vi "uSubscription IsAlive.vi"(8 "error in (no error)":errorcluster, 11 "uSubscription in":refnum<class "uSubscription.lvclass">) -> (0 "error out":errorcluster, 2 "Is Alive?":bool)   [LabVIEW 2023, in "uLib.lvlib" / "uSubscription.lvclass"]
uses:
  uSubscription.lvclass
  uSubscription.lvclass/uSubscription.ctl
  uTransport/uTransport/uTransport.lvclass
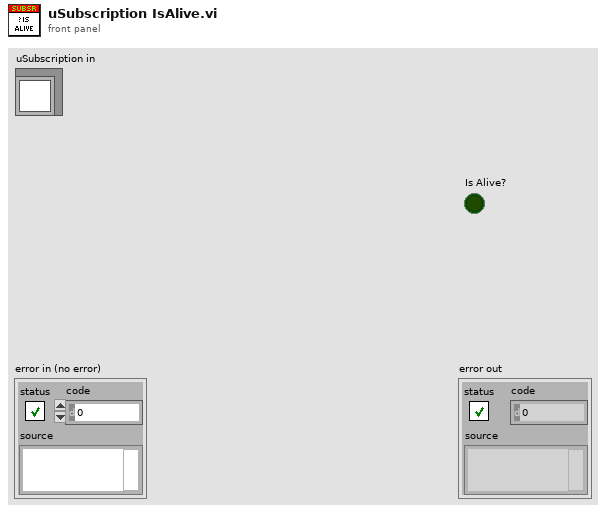
[diagram p1: front panel]
types:
  T1 = typedef "uLib.lvlib/uSubscription.lvclass/TypeDef_uSubscriptionPrivateData.ctl" = cluster{"Destination CMD":string, "uNotifyMode":refnum<class "uNotifyMode.lvclass">, "Destination uTransport":refnum<class "uTransport.lvclass">}
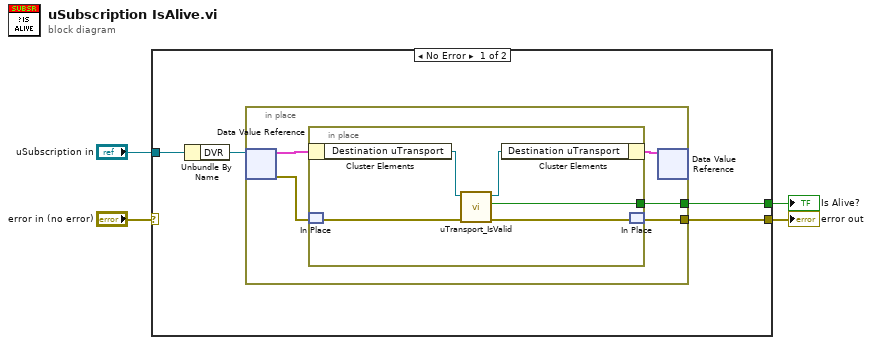
[diagram p0: block diagram]
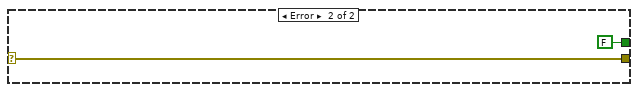
[diagram p2: hidden frame]
diagram:
  n1 = case shown="No Error" "error in (no error)" {
    selector: "error in (no error)" -> [_ w20]
    tunnel: [w8 w20] -> w4
    tunnel: [w7 FALSE ("IsValid?")] -> w3
    tunnel: "uSubscription in" -> [w6 _]
    frame No Error {
      n2 = Unbundle By Name(w6) -> ("DVR"=w5:refnum<data-value>)
      n3 = in-place {
        in-place-border: [w10] -> w8
        in-place-border: [w13] -> w7
        n4 = in-place-dvr #1(w5) -> (w12:T1, w11:errorcluster)
        n5 = in-place {
          in-place-border: [w18] -> w13
          n6 = in-place-cluster #2(w12) -> ("Destination uTransport"=w16:refnum<class "uTransport.lvclass">)
          n7 = in-place-match #3(w11) -> (w15:errorcluster)
          n8 = call-dynamic "uTransport_IsValid.vi"("error in (no error)"=w15, "uTransport in"=w16) -> ("error out"=w14:errorcluster, "IsValid?"=w18:bool, "uTransport out"=w17:refnum<class "uTransport.lvclass">)  [unwired: 7 in]
          n9 = in-place-cluster #2("Destination uTransport"=w17) -> (w9:T1)
          n10 = in-place-match #3(w14) -> (w10:errorcluster)
        }
        n11 = in-place-dvr #1(w9) -> ()  [unwired: 2 out]
      }
    }
    frame Error {
    }
  }
  "error out" <- w4
  "Is Alive?" <- w3
